vi "Bank.vi"() -> ()   [LabVIEW 2010]
doc: "This VI simulates the transactions that occur in a bank and demonstrates race conditions.\n\nRun the VI, and attempt a simultaneous transaction and notice that either the withdrawal or deposit is lost. Try to find and solve the problem."
panel:
  out "Balance":dbl
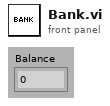
[diagram p1: front panel]
types:
  T1 = typedef "Account Info.ctl" = cluster{"Bank Rendezvous":T2, "Withdrawal Queue":refnum<queue>, "Deposit Queue":refnum<queue>}
  T2 = typedef "Rendezvous RefNum" = refnum<k1>
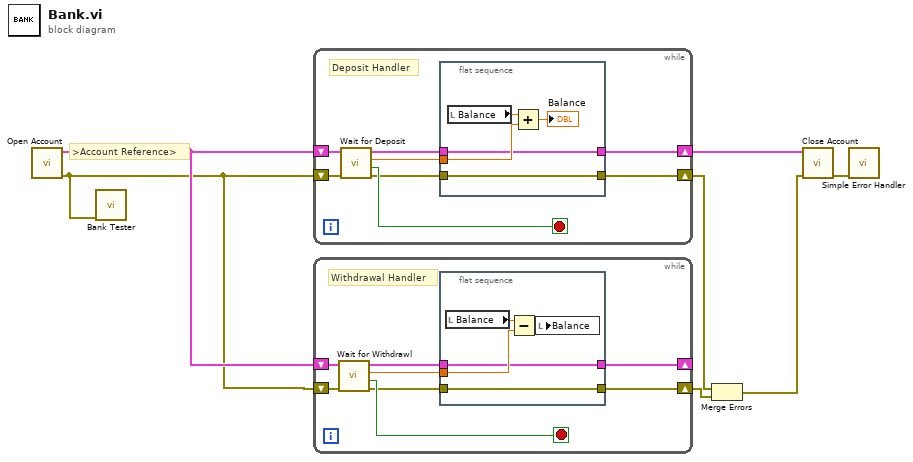
[diagram p0: block diagram]
diagram:
  # ">Account Reference>"
  n1 = call "Open Account.vi"() -> ("error out"=w1:errorcluster, "Account info"=w7:T1)  [unwired: 10 in]
  n2 = call "Bank Tester.vi"("error in (no error)"=w1) -> ()  [unwired: 10 in, 1 out]
  n3 = while {
    shift-right: [w11] -> w4
    shift-left: w7 -> [w14]
    shift-right: [w8] -> w6
    shift-left: w1 -> [w13]
    stop <- w10 stop-if-true
    # "Deposit Handler"
    n4 = call "Wait for Deposit.vi"("error in (no error)"=w13, "Account info"=w14) -> ("error out"=w9:errorcluster, "Stop?"=w10:bool, "Deposit Amount"=w15:dbl, "Account info out"=w12:T1)  [unwired: 6 in]
    n5 = flat-sequence {
      tunnel: w15 -> [w20]
      tunnel: [w17] -> w11
      tunnel: w12 -> [w17]
      tunnel: w9 -> [w16]
      tunnel: [w16] -> w8
      frame #0 {
        n6 = local read "Balance"() -> (w18:dbl)
        n7 = Add(x=w18, y=w20) -> (x+y=→"Balance":dbl)
      }
    }
  }
  n8 = while {
    shift-right: [w24] -> _
    shift-left: w7 -> [w27]
    shift-right: [w21] -> w5
    shift-left: w1 -> [w26]
    stop <- w23 stop-if-true
    # "Withdrawal Handler"
    n9 = call "Wait for Withdrawl.vi"("error in (no error)"=w26, "Account info"=w27) -> ("error out"=w22:errorcluster, "Stop?"=w23:bool, "Withdrawal Amount"=w28:dbl, "Account info out"=w25:T1)  [unwired: 6 in]
    n10 = flat-sequence {
      tunnel: w28 -> [w31]
      tunnel: w25 -> [w30]
      tunnel: w22 -> [w29]
      tunnel: [w30] -> w24
      tunnel: [w29] -> w21
      frame #0 {
        n11 = local read "Balance"() -> (w32:dbl)
        n12 = Subtract(x=w32, y=w31) -> (x-y=w33:dbl)
        n13 = local write "Balance"(w33) -> ()
      }
    }
  }
  n14 = Merge Errors(w6, w5) -> (w2:errorcluster)
  n15 = call "Close Account.vi"("error in"=w2, "Account info"=w4) -> ("error out"=w3:errorcluster)  [unwired: 9 in]
  n16 = call <vilib>:"Simple Error Handler.vi"("error in (no error)"=w3) -> ()  [unwired: 4 in, 5 out]
